vi "formula node.vi"() -> ()   [LabVIEW 2017]
panel:
  out "output variable 2":dbl
  out "output variable":dbl
  in  "X2":dbl
  in  "X1":dbl
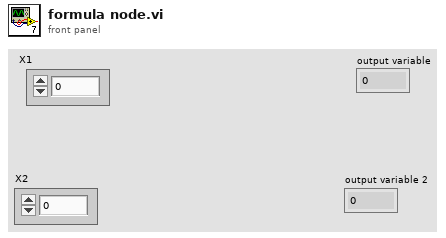
[diagram p1: front panel]
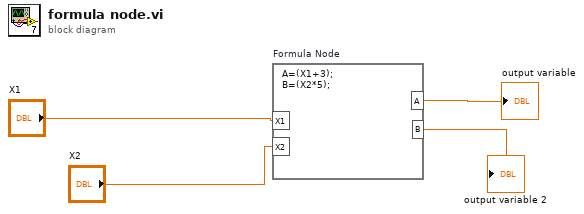
[diagram p0: block diagram]
diagram:
  n1 = formula code="A=(X1+3);\nB=(X2*5);"("X1"="X1", "X2"="X2") -> ("A"=→"output variable":dbl, "B"=→"output variable 2":dbl)
